vi "Manage Escalation Time.vi"(8 "error in (no error)":errorcluster) -> (0 "error out":errorcluster)   [LabVIEW 2017]
uses:
  <vilib>/Utility/miscctls.llb/LVRowAndColumnTypeDef.ctl
  <vilib>/Utility/miscctls.llb/LVBoundsTypeDef.ctl
panel:
  in  "Table":string[][](table)
  in  "Save":bool
  # "Manage Escalation Time"
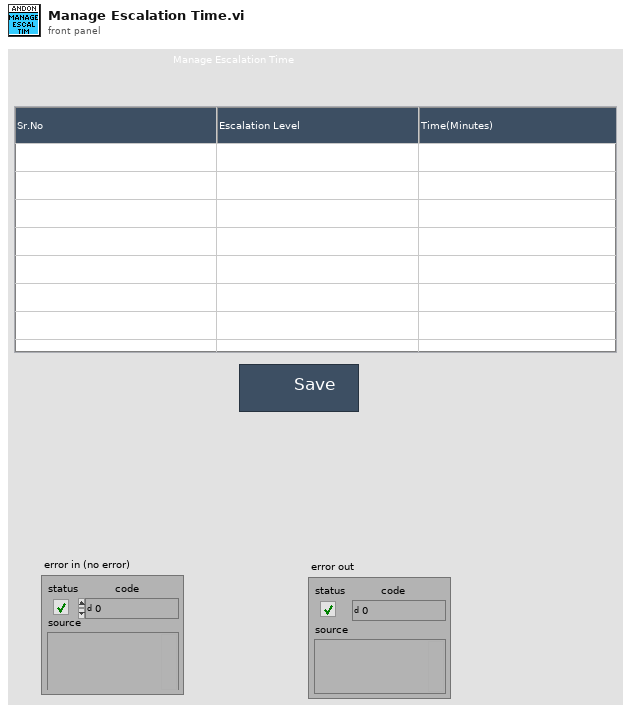
[diagram p1: front panel]
types:
  T1 = typedef "LVBoundsTypeDef.ctl" = cluster{"Width":u32, "Height":u32}
  T2 = typedef "LVRowAndColumnTypeDef.ctl" = cluster{"Row":i32, "Column":i32}
  T3 = enum32{"invalid app kind", "Development System", "Run Time System", "Student Edition", "Embedded LabVIEW", "Evaluation", "Custom"}
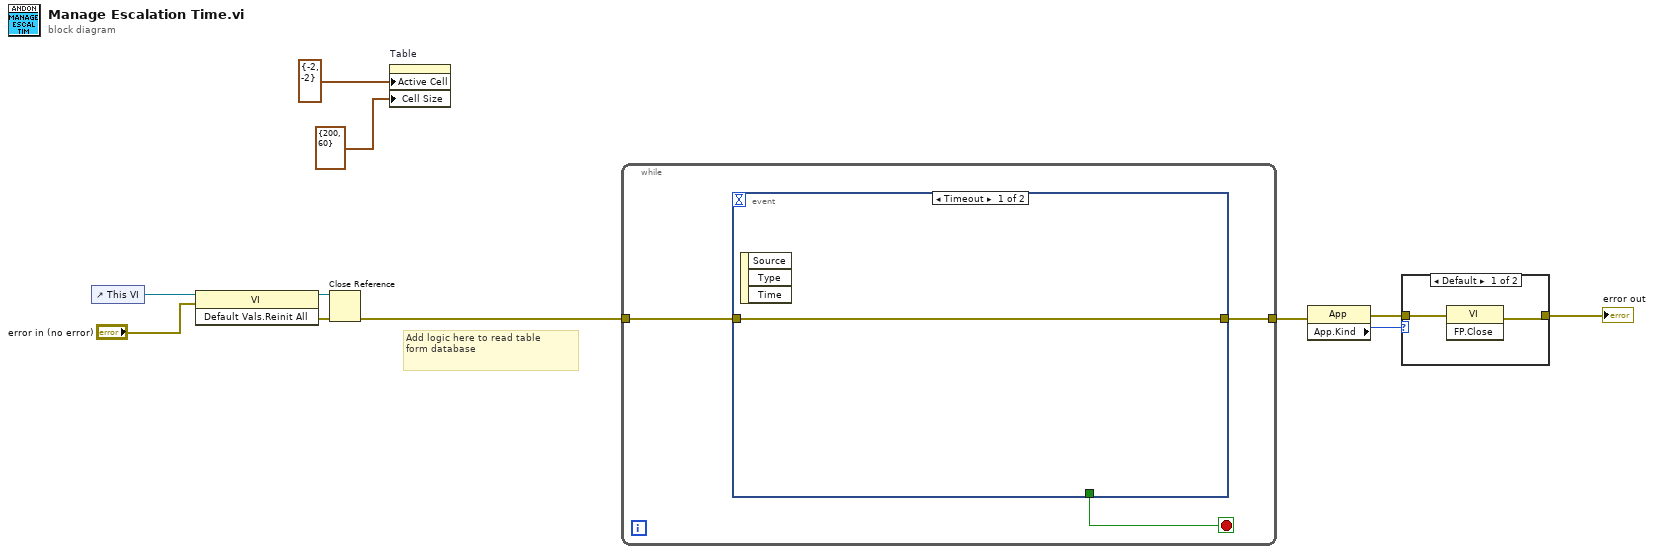
[diagram p0: block diagram]
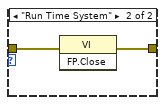
[diagram p2: hidden frame]
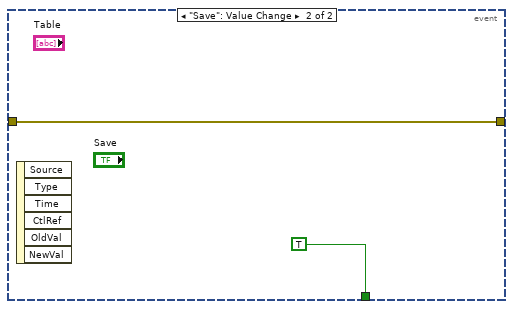
[diagram p3: hidden frame]
diagram:
  # "Add logic here to read table\nform database"
  n1 = control-ref of="This VI"() -> (w9:refnum<vi>)
  n2 = invoke class="VI" method="Default Vals.Reinit All"(reference=w9, error in="error in (no error)") -> (reference out=w6:refnum<vi>, error out=w7:errorcluster)  [unwired: 1 in, 1 out]
  n3 = Close Reference(reference=w6, error in (no error)=w7) -> (error out=w5:errorcluster)
  n4 = property on="Table" class="Tbl (strict)"("Active Cell"=T2 {"Row"=-2, "Column"=-2} ("Active Cell:Active Cell"), "Cell Size"=T1 {"Width"=200, "Height"=60} ("Active Cell:Cell Size")) -> ()  [unwired: 2 in, 2 out]
  n5 = while {
    tunnel: w5 -> [w14]
    tunnel: [w13] -> w1
    stop <- w12 stop-if-true
    n6 = event shown="[0] Timeout" {
      selector: _ -> [_ _]
      dyn-events: _ -> [_ _]
      timeout: _ -> [_ _]
      tunnel: w14 -> [w15 w17]
      tunnel: [w15 w17] -> w13
      tunnel: [_ TRUE] -> w12
      event Timeout {
        n7 = event-data() -> ()  [unwired: 1 in, 3 out]
      }
      event "Save": Value Change {
        n8 = event-data() -> ()  [unwired: 1 in, 6 out]
      }
    }
  }
  n9 = property class="App"(error in=w1) -> (error out=w3:errorcluster, "App.Kind"=w4:T3)  [unwired: 1 in, 1 out]
  n10 = case shown="Default" w4 {
    tunnel: w3 -> [w19 w21]
    tunnel: [w18 w20] -> w2
    frame Default {
      n11 = invoke class="VI" method="FP.Close"(error in=w19) -> (error out=w18:errorcluster)  [unwired: 2 in, 2 out]
    }
    frame "Run Time System" {
      n12 = invoke class="VI" method="FP.Close"(error in=w21) -> (error out=w20:errorcluster)  [unwired: 2 in, 2 out]
    }
  }
  "error out" <- w2
